vi "Load Data.vi"(8 "error in (no error)":errorcluster, 10 "JSON Data":string, 11 "VI Reference":refnum<vi>) -> (0 "error out":errorcluster, 3 "VI Refnum out":refnum<vi>)   [LabVIEW 2017, in "LVUnit Test Case.lvclass"]
doc: "Prepares the specified test case for execution."
uses:
  LVUnit Test Case.lvclass
  <vilib>/PNR/JSONtext Object Serialization/Generic Object Serializer/Generic Object Serializer.lvclass
  C:/Program Files/National Instruments/LabVIEW 2017/vi.lib/JDP Science/JSONtext/LVClass Serializer/JSONtext LVClass Serializer.lvclass
  <vilib>/PNR/JSONtext Object Serialization/Generic Object Serializer/Type Name Handling.ctl
  <vilib>/PNR/JSONtext Object Serialization/Generic Object Serializer/Generic Object Serializer.lvclass/Generic Object Serializer.ctl
  bede4881-c3ee-429c-a29f-335cd5e8a060.vi
  <vilib>/PNR/JSONtext Object Serialization/Generic Object Serializer/Write Type Name Handling.vi
  <vilib>/JDP Science/JSONtext/Find Item.vi
  <vilib>/JDP Science/JSONtext/Next JSON Value.vi
  <vilib>/JDP Science/JSONtext/String Subset.vi
  <vilib>/JDP Science/JSONtext/Parsing/Advance past next JSON Value (inlined COPY).vi
  <vilib>/JDP Science/JSONtext/Parsing/Advance past whitespace.vi
  <vilib>/JDP Science/JSONtext/Parsing/Advance past String.vi
  <vilib>/JDP Science/JSONtext/Parsing/Advance past Number.vi
  <vilib>/JDP Science/JSONtext/Parsing/Advance past Line Ending.vi
  <vilib>/JDP Science/JSONtext/Parsing/Parse Full Path or Item Name.vi
  <vilib>/JDP Science/JSONtext/Parsing/Advance past Array.vi
  <vilib>/JDP Science/JSONtext/Parsing/Advance past Object.vi
  <vilib>/JDP Science/JSONtext/support/Error Cluster From Code.vi
  <vilib>/JDP Science/JSONtext/Offset/Find Item Locations by Path.vi
  <vilib>/JDP Science/JSONtext/JSON text to Variant.vi
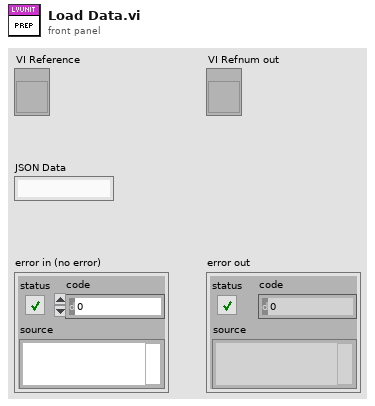
[diagram p1: front panel]
types:
  T1 = typedef "Generic Object Serializer.lvclass/Type Name Handling.ctl" = enum16{"None", "Inline"}
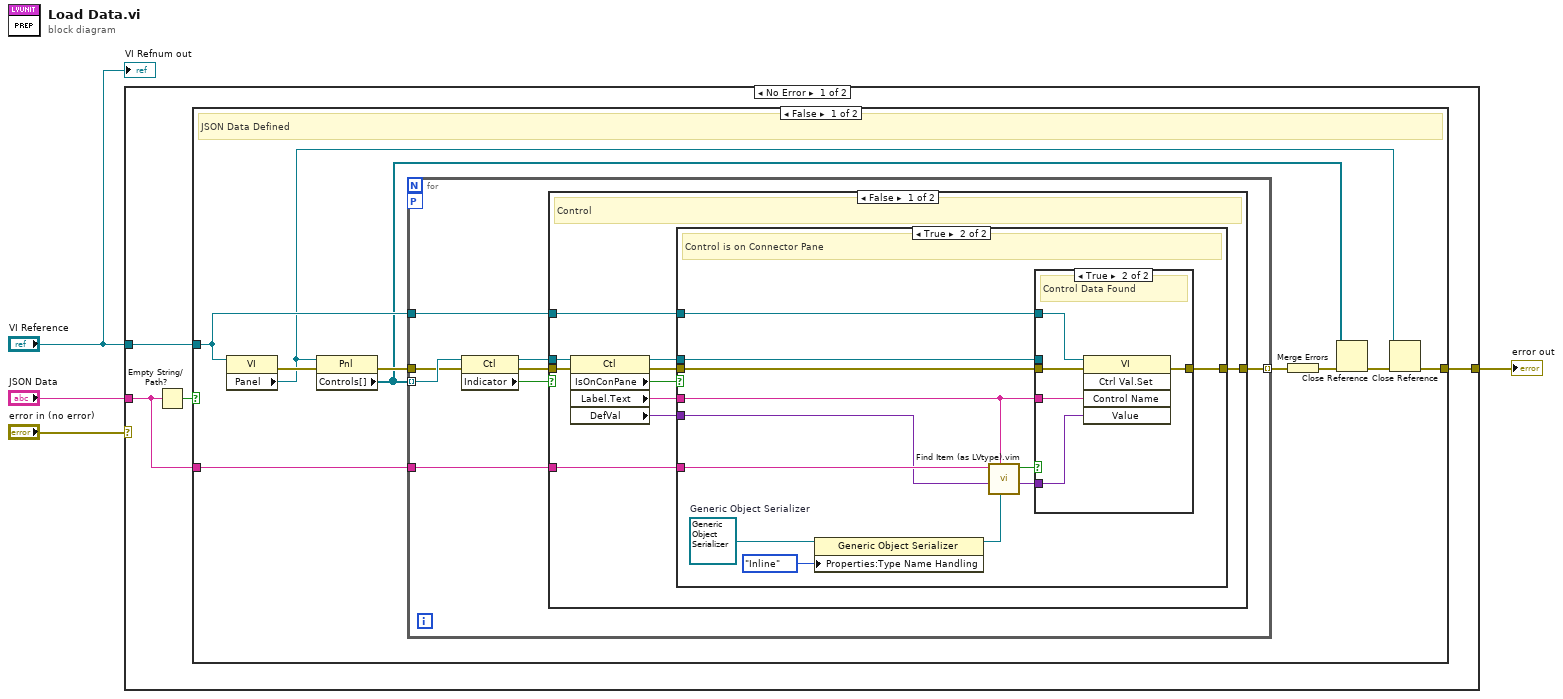
[diagram p0: block diagram]
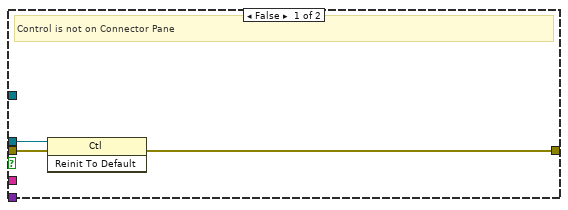
[diagram p2: hidden frame]
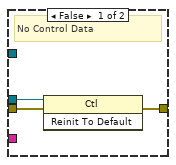
[diagram p3: hidden frame]
diagram:
  n1 = case shown="No Error" "error in (no error)" {
    selector: "error in (no error)" -> [_ w61]
    tunnel: [w8 w61] -> w4
    tunnel: "JSON Data" -> [w6 _]
    tunnel: "VI Reference" -> [w5 _]
    frame No Error {
      n2 = Empty String/Path?(string/path=w6) -> (empty?=w7:bool)
      n3 = case shown="False" w7 {
        tunnel: [w11 _] -> w8
        tunnel: w5 -> [w17 _]
        tunnel: w6 -> [w16 _]
        frame False {
          # "JSON Data Defined"
          n4 = property class="VI"(reference=w17) -> (error out=w15:errorcluster, "Panel"=w10:refnum<vi>)  [unwired: 1 in, 1 out]
          n5 = property class="Pnl"(reference=w10, error in=w15) -> (error out=w14:errorcluster, "Controls[]"=w12:refnum<vi>[])  [unwired: 1 out]
          n6 = for {
            tunnel: w17 -> [w25]
            tunnel: w16 -> [w26]
            tunnel: w12 -> [w23] mode=indexing
            tunnel: w14 -> [w22]
            tunnel: [w24] -> w18 mode=indexing
            workers-P: _ -> [_]
            n7 = property class="Ctl"(reference=w23, error in=w22) -> (reference out=w21:refnum<vi>, error out=w20:errorcluster, "Indicator"=w19:bool)
            n8 = case shown="False" w19 {
              tunnel: w26 -> [w34 _]
              tunnel: w25 -> [w31 _]
              tunnel: [w30 w60] -> w24
              tunnel: w21 -> [w29 _]
              tunnel: w20 -> [w28 w60]
              frame False {
                # "Control"
                n9 = property class="Ctl"(reference=w29, error in=w28) -> (reference out=w32:refnum<vi>, error out=w35:errorcluster, "IsOnConPane"=w36:bool, "Label.Text"=w33:string, "DefVal"=w27:variant)
                n10 = case shown="True" w36 {
                  tunnel: [w38 w49] -> w30
                  tunnel: w35 -> [w39 w51]
                  tunnel: w34 -> [_ w48]
                  tunnel: w33 -> [_ w40]
                  tunnel: w32 -> [w37 w44]
                  tunnel: w31 -> [_ w50]
                  tunnel: w27 -> [_ w47]
                  frame False {
                    # "Control is not on Connector Pane"
                    n11 = invoke class="Ctl" method="Reinit To Default"(reference=w37, error in=w39) -> (error out=w38:errorcluster)  [unwired: 1 in, 2 out]
                  }
                  frame True {
                    w43 = refnum<class "Generic Object Serializer.lvclass"> refnum  # Generic Object Serializer
                    # "Control is on Connector Pane"
                    n12 = property class="Generic Object Serializer"(reference=w43, "Properties:Type Name Handling"=Type_Name_Handling."Inline" ("Type Name Handling")) -> (reference out=w42:refnum<class "Generic Object Serializer.lvclass">)  [unwired: 1 in, 1 out]
                    n13 = call "Find Item (as LVtype).vim"("LVClass Serializer"=w42, "$Path or Item Name"=w40, "Data Type and Default Value"=w47, "JSON"=w48) -> ("Data"=w46:variant, "Found"=w45:bool)  [unwired: 4 in, 2 out]
                    n14 = case shown="True" w45 {
                      tunnel: w51 -> [w54 w59]
                      tunnel: w50 -> [_ w58]
                      tunnel: [w53 w57] -> w49
                      tunnel: w40 -> [_ w56]
                      tunnel: w46 -> [_ w55]
                      tunnel: w44 -> [w52 _]
                      frame False {
                        # "No Control Data"
                        n15 = invoke class="Ctl" method="Reinit To Default"(reference=w52, error in=w54) -> (error out=w53:errorcluster)  [unwired: 1 in, 2 out]
                      }
                      frame True {
                        # "Control Data Found"
                        n16 = invoke class="VI" method="Ctrl Val.Set"(reference=w58, error in=w59, "Control Name"=w56, "Value"=w55) -> (error out=w57:errorcluster)  [unwired: 1 in, 4 out]
                      }
                    }
                  }
                }
              }
              frame True {
                # "Indicator"
              }
            }
          }
          n17 = Merge Errors(w18) -> (w9:errorcluster)
          n18 = Close Reference(reference=w12, error in (no error)=w9) -> (error out=w13:errorcluster)
          n19 = Close Reference(reference=w10, error in (no error)=w13) -> (error out=w11:errorcluster)
        }
        frame True {
          # "No JSON Data"
        }
      }
    }
    frame Error {
    }
  }
  "error out" <- w4
  "VI Refnum out" <- "VI Reference"
